vi "Create Log File.vi"(8 "error in":errorcluster, 11 "Sys Log in":refnum<class "System Log.lvclass">) -> (0 "error out":errorcluster, 3 "Sys Log out":refnum<class "System Log.lvclass">)   [LabVIEW 2014, in "System Log.lvclass"]
uses:
  System Log.lvclass
  System Log.lvclass/System Log.ctl
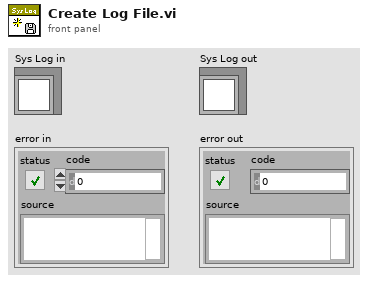
[diagram p1: front panel]
types:
  T1 = enum16{"open", "replace", "create", "open or create", "replace or create", "replace or create with confirmation"}
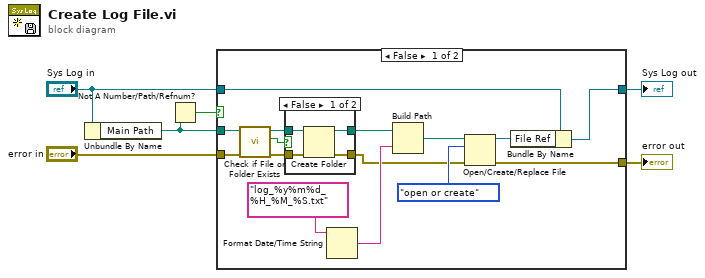
[diagram p0: block diagram]
diagram:
  n1 = Unbundle By Name("Sys Log in") -> ("Main Path"=w6:path)
  n2 = Not A Number/Path/Refnum?(number/path/refnum=w6) -> (NaN/Path/Refnum?=w1:bool)
  n3 = case shown="False" w1 {
    tunnel: "Sys Log in" -> [w21 w29]
    tunnel: [w20 w29] -> w3
    tunnel: "error in" -> [w14 w28]
    tunnel: [w18 w28] -> w5
    tunnel: w6 -> [w15 _]
    frame False {
      n4 = call <vilib>:"Check if File or Folder Exists.vi"("error in (no error)"=w14, "path"=w15) -> ("error out"=w11:errorcluster, "file or folder exists?"=w13:bool, "dup path"=w12:path)  [unwired: 7 in]
      n5 = case shown="False" w13 {
        tunnel: w12 -> [w25 w27]
        tunnel: w11 -> [w24 w26]
        tunnel: [w23 w27] -> w10
        tunnel: [w22 w26] -> w7
        frame False {
          n6 = Create Folder(path (use dialog)=w25, error in=w24) -> (created path=w23:path, error out=w22:errorcluster)  [unwired: 1 in, 1 out]
        }
        frame True {
        }
      }
      n7 = Format Date/Time String(time format string (%c)="log_%y%m%d_%H_%M_%S.txt") -> (date/time string=w9:string)  [unwired: 2 in]
      n8 = Build Path(base path=w10, name or relative path=w9) -> (appended path=w8:path)
      n9 = Open/Create/Replace File(file path (use dialog)=w8, error in=w7, operation (0:open)=T1."open or create") -> (refnum out=w19:refnum<file>, error out=w18:errorcluster)  [unwired: 3 in, 1 out]
      n10 = Bundle By Name(cluster=w21, "File Ref"=w19) -> (w20:refnum<class "System Log.lvclass">)
    }
    frame True {
    }
  }
  "error out" <- w5
  "Sys Log out" <- w3
